vi "Telescope Deg Min Sec to Angle.vi"(11 "deg min sec":dbl[](array[numeric])) -> (3 "result":dbl)   [LabVIEW 2022 SP3, in "Telescope.lvclass"]
uses:
  Telescope.lvclass
  Telescope.lvclass/Telescope.ctl
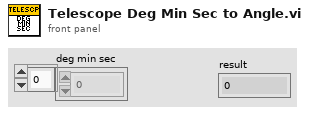
[diagram p1: front panel]
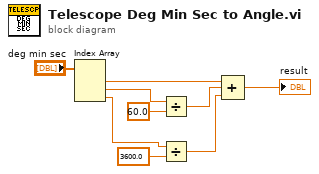
[diagram p0: block diagram]
diagram:
  n1 = Index Array(array="deg min sec") -> (element #1=w9:dbl, element #2=w8:dbl, element #3=w5:dbl)  [unwired: 3 in]
  n2 = Divide(x=w8, y=60.0) -> (x/y=w3:dbl)
  n3 = Divide(x=w5, y=3600.0) -> (x/y=w4:dbl)
  n4 = Compound Arithmetic op=ADD(w9, w3, w4) -> (→"result":dbl)
